vi "Factorial_Shift_Register.vi"() -> ()   [LabVIEW 2017]
panel:
  out "Factorial of N":i32
  in  "N":i32
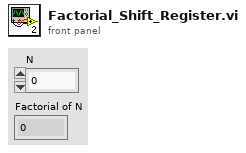
[diagram p1: front panel]
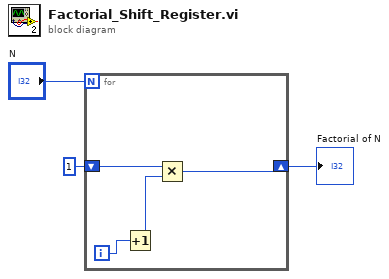
[diagram p0: block diagram]
diagram:
  n1 = for {
    N: "N" -> [_]
    shift-right: [w6] -> w2
    shift-left: 1 -> [w7]
    i -> [w5]
    n2 = Increment(x=w5) -> (x+1=w4:i32)
    n3 = Multiply(x=w7, y=w4) -> (x*y=w6:i32)
  }
  "Factorial of N" <- w2
